vi "ReadMaxAmp.vi"(8 "error in (no error)":errorcluster, 9 "Channel":dbl, 11 "Scope In":refnum<class "Scope.lvclass">) -> (0 "error out":errorcluster, 1 "Amplitude":dbl, 3 "Scope Out":refnum<class "Scope.lvclass">)   [LabVIEW 2019, in "Scope.lvclass"]
uses:
  Scope.lvclass
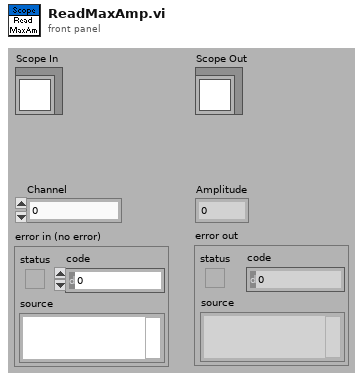
[diagram p1: front panel]
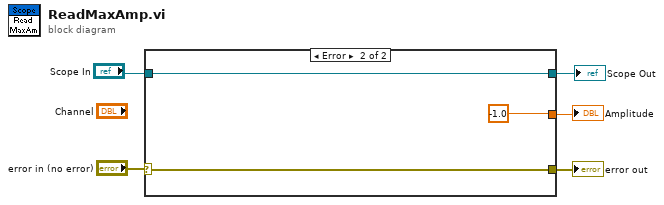
[diagram p0: block diagram]
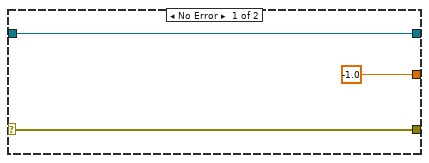
[diagram p2: hidden frame]
diagram:
  n1 = case shown="Error" "error in (no error)" {
    selector: "error in (no error)" -> [w6 w11]
    tunnel: [w6 w11] -> w5
    tunnel: [w8 w10] -> w1
    tunnel: "Scope In" -> [w8 w10]
    tunnel: [-1.0 -1.0] -> w3
    frame No Error {
    }
    frame Error {
    }
  }
  "error out" <- w5
  "Amplitude" <- w3
  "Scope Out" <- w1
